vi "LVClass_Pupil dtor.vi"(0 "Pupil in":refnum<class "Pupil.lvclass">, 11 "error in (no error)":errorcluster) -> (4 "Pupil out":refnum<class "Pupil.lvclass">, 15 "error out":errorcluster)   [LabVIEW 2020, in "Pupil.lvclass"]
doc: "Pupil destructor.\n\n--------------------------------------------------------------------------------\n\n<B>PupilIn </B> : Pupil object.\n<B>PupilOut </B> : Pupil object.\n<B>ErrorIn </B> : Error\n<B>ErrorOut </B> : Error\n\n--------------------------------------------------------------------------------"
uses:
  Pupil.lvclass
  Pupil.lvclass/Pupil.ctl
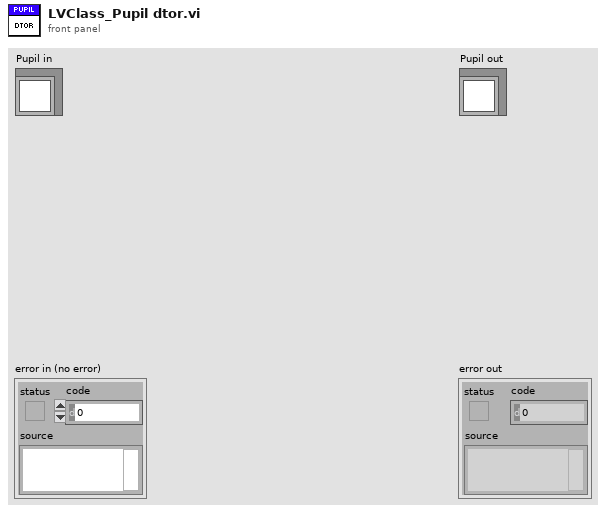
[diagram p1: front panel]
types:
  T1 = typedef "Handle creation.ctl" = enum16{"By ctor", "By write function"}
  T2 = typedef "ClassID.ctl" = i64
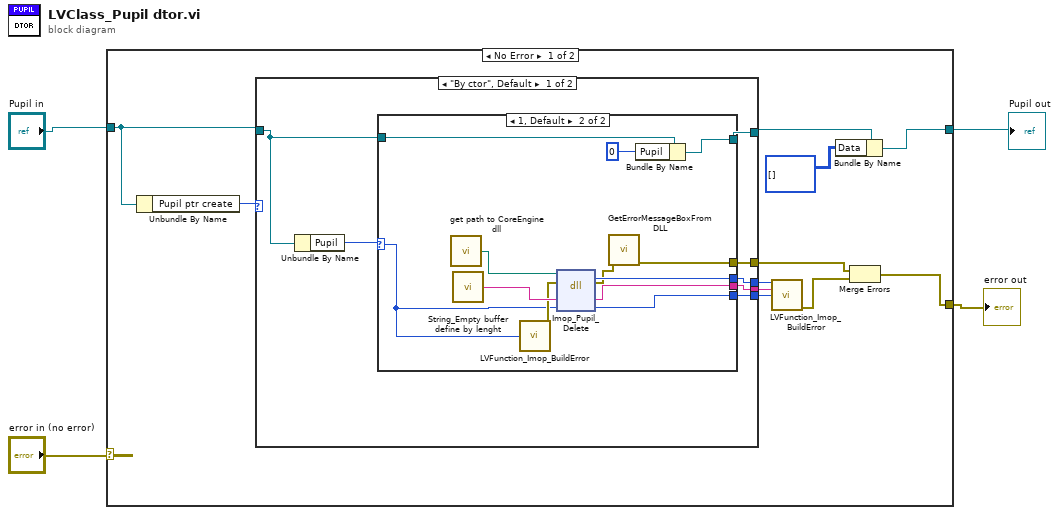
[diagram p0: block diagram]
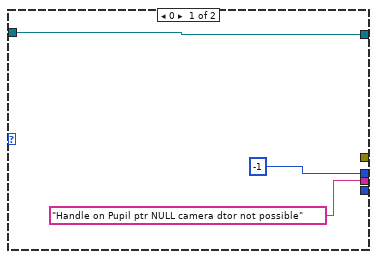
[diagram p2: hidden frame]
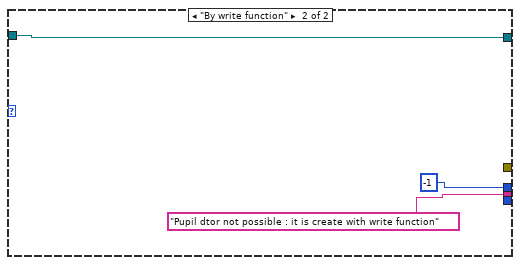
[diagram p3: hidden frame]
diagram:
  n1 = case shown="No Error" "error in (no error)" {
    selector: "error in (no error)" -> [_ w40]
    tunnel: "Pupil in" -> [w13 w41]
    tunnel: [w7 w41] -> w1
    tunnel: [w10 w40] -> w2
    frame No Error {
      n2 = Unbundle By Name(w13) -> ("Pupil ptr create"=w12:T1)
      n3 = case shown="\"By ctor\", Default" w12 {
        tunnel: [w22 "Pupil dtor not possible : it is create with write function" ("message")] -> w15
        tunnel: [w21 -1] -> w14
        tunnel: w13 -> [w19 w39]
        tunnel: [w20 w39] -> w8
        tunnel: [w17 _] -> w9
        tunnel: [w16 _] -> w5
        frame "By ctor", Default {
          n4 = Unbundle By Name(w19) -> ("Pupil"=w18:T2)
          n5 = case shown="1, Default" w18 {
            selector: w18 -> [_ w26]
            tunnel: ["Handle on Pupil ptr NULL camera dtor not possible" ("message") w35] -> w22
            tunnel: [-1 w34] -> w21
            tunnel: w19 -> [w23 w30]
            tunnel: [w23 w29] -> w20
            tunnel: [_ w28] -> w17
            tunnel: [_ w26] -> w16
            frame 0 {
            }
            frame 1, Default {
              n6 = call "get path to CoreEngine dll.vi"() -> ("path to wavekit library"=w33:path)  [unwired: 14 in, 1 out]
              n7 = call "String_Empty buffer define by lenght.vi"() -> ("Empty buffer"=w36:string)  [unwired: 1 in]
              n8 = call "LVFunction_Imop_BuildError.vi"("Adresse"=w26) -> ("error out"=w27:errorcluster)  [unwired: 14 in]
              n9 = dll-call lib="D:/soft/HASO_v3/SVN_trunk/ImOpCoreEngine4_LV2011/DLLs/c_interface_vc100.dll" fn="Imop_Pupil_Delete"(path in=w33, error in=w27, "message"=w36, "objet"=w26) -> (error out=w32:errorcluster, "return type"=w34:i32, "message"=w35:string)  [unwired: 2 in, 1 out]
              n10 = call "GetErrorMessageBoxFromDLL.vi"("error IN"=w32) -> ("error OUT"=w28:errorcluster)  [unwired: 10 in]
              n11 = Bundle By Name(cluster=w30, "Pupil"=u32 0) -> (w29:refnum<class "Pupil.lvclass">)
            }
          }
        }
        frame "By write function" {
        }
      }
      n12 = call "LVFunction_Imop_BuildError.vi"("code"=w14, "String to Prepend to source (\"\")"=w15, "Adresse"=w5) -> ("error out"=w11:errorcluster)  [unwired: 12 in]
      n13 = Bundle By Name(cluster=w8, "Data"=i32[][] []) -> (w7:refnum<class "Pupil.lvclass">)
      n14 = Merge Errors(w9, w11) -> (w10:errorcluster)
    }
    frame Error {
    }
  }
  "error out" <- w2
  "Pupil out" <- w1
